vi "Open Generic Property.vi"(0 "SLSC Local in":refnum<class "SLSC Local.lvclass">, 5 "resource":string, 7 "property in":refnum<k21>, 11 "error in (no error)":errorcluster) -> (4 "SLSC Local out":refnum<class "SLSC Local.lvclass">, 8 "property out":refnum<k21>, 15 "error out":errorcluster)   [LabVIEW 2015, in "SLSC Interfaces.lvlib" / "SLSC Local.lvclass"]
uses:
  SLSC Local.lvclass
  <vilib>/SLSC/SLSC.lvlib
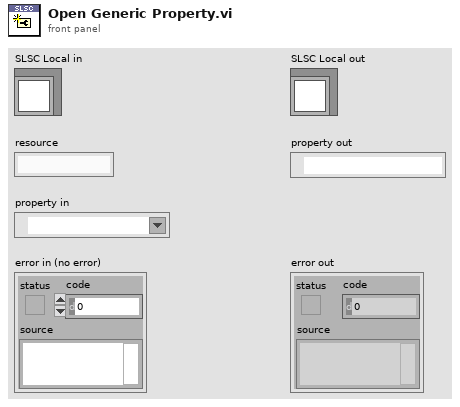
[diagram p1: front panel]
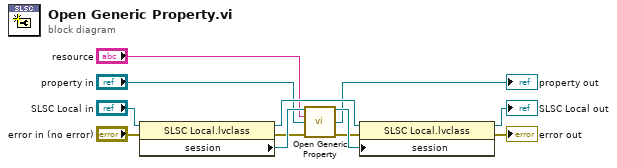
[diagram p0: block diagram]
diagram:
  n1 = property class="SLSC Local.lvclass"(reference="SLSC Local in", error in="error in (no error)") -> (reference out=w12:refnum<class "SLSC Local.lvclass">, error out=w6:errorcluster, "session"=w11:refnum<k21>)
  n2 = call <vilib>:"Open Generic Property.vi"("session in"=w11, "resource"="resource", "property in"="property in", "error in (no error)"=w6) -> ("session out"=w10:refnum<k21>, "property out"=→"property out":refnum<k21>, "error out"=w4:errorcluster)  [unwired: 9 in]
  n3 = property class="SLSC Local.lvclass"(reference=w12, error in=w4, "session"=w10) -> (reference out=→"SLSC Local out":refnum<class "SLSC Local.lvclass">, error out=→"error out":errorcluster)
